vi "register_for_event_auth.vi"(8 "error in (no error)":errorcluster) -> (0 "error out":errorcluster, 3 "event_registration":refnum<event-registration>)   [LabVIEW 2015, in "lv-dropbox-examples.lvlib"]
uses:
  lv-dropbox-examples.lvlib
  _controls/authorization_response.ctl
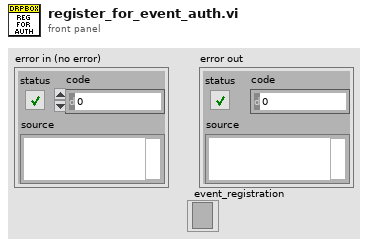
[diagram p1: front panel]
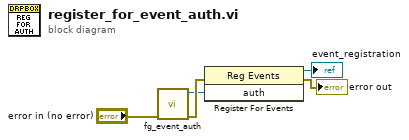
[diagram p0: block diagram]
diagram:
  n1 = call "fg_event_auth.vi"("error in (no error)"="error in (no error)") -> ("error out"=w4:errorcluster, "auth"=w2:refnum<user-event>)  [unwired: 9 in]
  n2 = register-events(error in=w4, w2) -> (reference out=→"event_registration":refnum<event-registration>, error out=→"error out":errorcluster)  [unwired: 1 in]
